vi "svx_DAQ_SaveTaskToMAX.vi"(8 "error in (no error)":errorcluster, 10 "Display State In":T2={"Channel Info Array"=[], "Timing Mode"=enum."Time", "Timing Control 1"=0.0, "Timing Control 2"=0.0, "Timing Control 3"=0, "Timing Indicator 1"=0.0, "Reference Visible?"=FALSE, "Reference Type"=enum."<none>", "Tachometer Channel"="", "Tach Pulses Per Rev"=0, "Tach Direction"=enum."CW", "Tach Slope"=enum."Rising", "Tach Threshold"=0.0, "Trigger Channel"="", "Trigger Level"=0.0, "Pretrigger Samples"=1, "Trigger Slope"=enum."Falling", "Trigger Hysteresis"=0.0, "Logging Visible?"=FALSE, "Enable Logging"=FALSE, "Logfile Path"=path "c:/test.tdms"} caption="State" {"Timing Control 2" format="%#_6f"; "Channel Info Array"."Max" min=0.0 format="± %^#_4g"; "Channel Info Array"."Channel Type" items=["Voltage (V)"=0, "Charge (C)"=9, "-"=99, "SPL (Pa)"=3, "Force (lbf)"=6, "Force (N)"=1, "Acceleration (g) - IEPE"=2, "Acceleration (g) - Charge"=12, "Acceleration (g) - 4 wire DC Voltage"=22, "Velocity (in/s)"=7, "Velocity (mm/s)"=8, "Prox Probe (mil)"=4, "Prox Probe (mm)"=5]}, 11 "Task In":T1) -> (0 "error out":errorcluster)   [LabVIEW 2017, in "SVX NI-DAQmx AI Configuration XControl.xctl"]
uses:
  <vilib>/addons/Sound and Vibration/svt_DAQmx/Configuration XControl/SVX NI-DAQmx AI Configuration XControl.xctl
  <vilib>/addons/Sound and Vibration/svt_DAQmx/Configuration XControl/SubVIs/svx_DAQ_State.ctl
  <vilib>/addons/Sound and Vibration/svt_DAQmx/Configuration XControl/Controls/svx_DAQ_ChannelInfo.ctl
  <vilib>/addons/Sound and Vibration/svt_DAQmx/Configuration XControl/Controls/svx_DAQ_ChannelType.ctl
  <vilib>/addons/Sound and Vibration/svt_DAQmx/Configuration XControl/Controls/svx_DAQ_Coupling.ctl
  <vilib>/addons/Sound and Vibration/svt_DAQmx/Configuration XControl/Controls/svx_DAQ_Excitation.ctl
  <vilib>/addons/Sound and Vibration/svt_DAQmx/Configuration XControl/Controls/svx_DAQ_TimingType.ctl
  <vilib>/addons/Sound and Vibration/svt_DAQmx/Configuration XControl/Controls/svx_DAQ_ReferenceType.ctl
  <vilib>/addons/Sound and Vibration/svt_DAQmx/Configuration XControl/Controls/svx_DAQ_RotationDirection.ctl
  <vilib>/addons/Sound and Vibration/svt_DAQmx/Configuration XControl/Controls/svx_DAQ_Tach_Slope.ctl
  <vilib>/addons/Sound and Vibration/svt_DAQmx/Configuration XControl/Controls/svx_DAQ_Trigger_Slope.ctl
  <vilib>/addons/Sound and Vibration/svt_DAQmx/Configuration XControl/SubVIs/svx_DAQ_Data.ctl
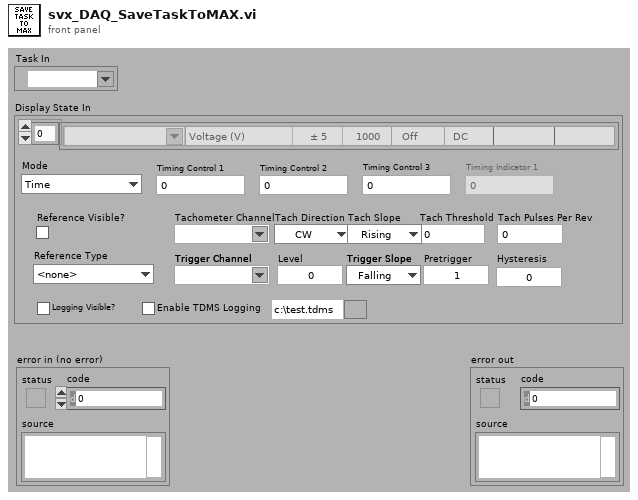
[diagram p1: front panel]
types:
  T1 = typedef "SVX NI-DAQmx AI Configuration XControl.xctl/svx_DAQ_Data.ctl" = refnum<k21>
  T2 = typedef "SVX NI-DAQmx AI Configuration XControl.xctl/svx_DAQ_State.ctl" = cluster{"Channel Info Array":T3[], "Timing Mode":T7, "Timing Control 1":dbl, "Timing Control 2":dbl, "Timing Control 3":i32, "Timing Indicator 1":dbl, "Reference Visible?":bool, "Reference Type":T8, "Tachometer Channel":string, "Tach Pulses Per Rev":i32, "Tach Direction":T9, "Tach Slope":T10, "Tach Threshold":dbl, "Trigger Channel":string, "Trigger Level":dbl, "Pretrigger Samples":i32, "Trigger Slope":T11, "Trigger Hysteresis":dbl, "Logging Visible?":bool, "Enable Logging":bool, "Logfile Path":path}
  T3 = typedef "SVX NI-DAQmx AI Configuration XControl.xctl/svx_DAQ_ChannelInfo.ctl" = cluster{"Initialized?":bool, "DAQmx Channel":tag, "Channel Type":T4, "Max":dbl, "Sensitivity":dbl, "Excitation":bool, "Coupling":T5, "Location":string, "Orientation":string, "excitation":T6}
  T4 = typedef "SVX NI-DAQmx AI Configuration XControl.xctl/svx_DAQ_ChannelType.ctl" = u16
  T5 = typedef "SVX NI-DAQmx AI Configuration XControl.xctl/svx_DAQ_Coupling.ctl" = enum16{"AC", "DC"}
  T6 = typedef "svx_DAQ_Excitation.ctl" = enum16{"Off", "Min", "Max"}
  T7 = typedef "SVX NI-DAQmx AI Configuration XControl.xctl/svx_DAQ_TimingType.ctl" = enum16{"Time", "Frequency", "Order"}
  T8 = typedef "SVX NI-DAQmx AI Configuration XControl.xctl/svx_DAQ_ReferenceType.ctl" = enum16{"<none>", "Analog Tachometer", "Analog SW Trigger"}
  T9 = typedef "SVX NI-DAQmx AI Configuration XControl.xctl/svx_DAQ_RotationDirection.ctl" = enum16{"CW", "CCW"}
  T10 = typedef "SVX NI-DAQmx AI Configuration XControl.xctl/svx_DAQ_Tach_Slope.ctl" = enum16{"Rising", "Falling"}
  T11 = typedef "SVX NI-DAQmx AI Configuration XControl.xctl/svx_DAQ_Trigger_Slope.ctl" = enum16{"Falling", "Rising"}
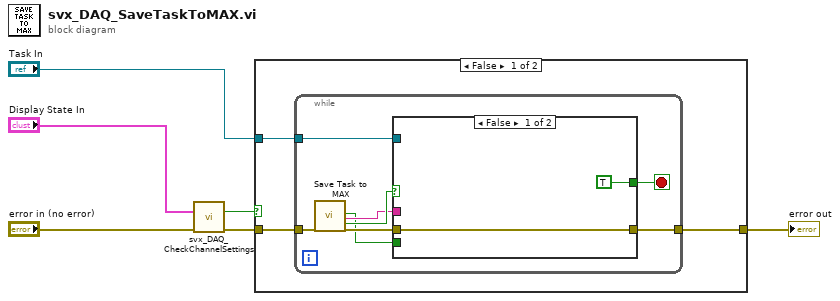
[diagram p0: block diagram]
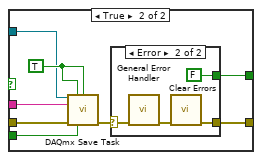
[diagram p2: hidden frame]
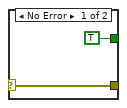
[diagram p3: hidden frame]
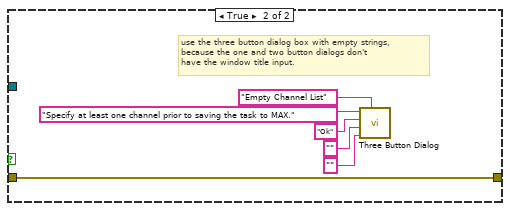
[diagram p4: hidden frame]
diagram:
  n1 = call <vilib>:"svx_DAQ_CheckChannelSettings.vi"("Display State In"="Display State In", "error in (no error)"="error in (no error)") -> ("Empty Channel List?"=w5:bool, "error out"=w4:errorcluster)  [unwired: 9 in, 3 out]
  n2 = case shown="False" w5 {
    tunnel: "Task In" -> [w9 _]
    tunnel: [w8 w39] -> w2
    tunnel: w4 -> [w7 w39]
    frame False {
      n3 = while {
        tunnel: w9 -> [w17]
        tunnel: [w16] -> w8
        tunnel: w7 -> [w14]
        stop <- w15 stop-if-true
        n4 = call "Save Task to MAX"("error in (no error)"=w14) -> ("Overwrite Existing Task?"=w10:bool, "Task Name"=w11:string, "OK"=w12:bool, "error out"=w13:errorcluster)  [unwired: 15 in]
        n5 = case shown="False" w12 {
          tunnel: w17 -> [_ w21]
          tunnel: [w19 w23] -> w16
          tunnel: w11 -> [_ w26]
          tunnel: w13 -> [w19 w25]
          tunnel: [TRUE w22] -> w15
          tunnel: w10 -> [_ w20]
          frame False {
          }
          frame True {
            w27 = TRUE ("allow interactive editing?")
            n6 = call <vilib>:"DAQmx Save Task.vi"("task/channels in"=w21, "allow interactive editing?"=w27, "allow interactive deletion?"=w27, "save as"=w26, "error in"=w25, "overwrite existing task?"=w20) -> ("error out"=w24:errorcluster)  [unwired: 8 in, 1 out]
            n7 = case shown="Error" w24 {
              selector: w24 -> [w29 w33]
              tunnel: [w29 w31] -> w23
              tunnel: [TRUE FALSE] -> w22
              frame No Error {
              }
              frame Error {
                n8 = call <vilib>:"General Error Handler.vi"("error in (no error)"=w33) -> ("error out"=w32:errorcluster)  [unwired: 10 in, 4 out]
                n9 = call <vilib>:"Clear Errors.vi"("error in (no error)"=w32) -> ("error out"=w31:errorcluster)  [unwired: 5 in, 1 out]
              }
            }
          }
        }
      }
    }
    frame True {
      # "use the three button dialog box with empty strings,\nbecause the one and two button dialogs don't\nhave the window title input."
      n10 = call <vilib>:"Three Button Dialog.vi"("Window Title (\"\")"="Empty Channel List" ("Message"), "Right Button Text (\"Cancel\")"="" ("Right Button Text (\"Cancel\")"), "Center Button Text (\"No\")"="" ("Center Button Text (\"No\")"), "Left Button Text (\"Yes\")"="Ok" ("Left Button Text (\"Yes\")"), "message"="Specify at least one channel prior to saving the task to MAX." ("Message")) -> ()  [unwired: 6 in, 1 out]
    }
  }
  "error out" <- w2
